vi "sub vi - password 1.vi"() -> (0 "RESULT":bool)   [LabVIEW 2013]
uses:
  program files/Global 1.vi
panel:
  in  "OK Button":bool
  in  "PASSWORD":string
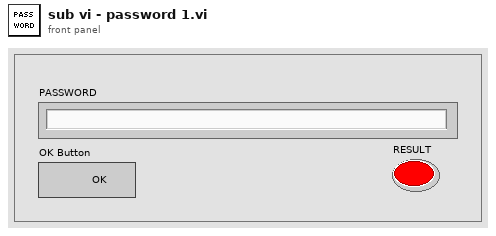
[diagram p1: front panel]
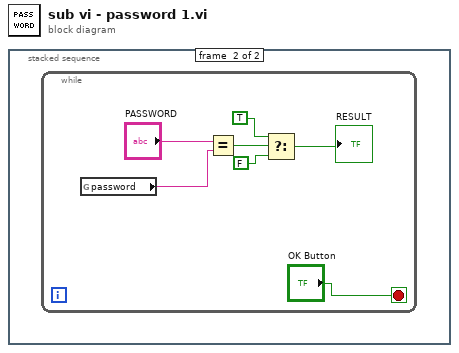
[diagram p0: block diagram]
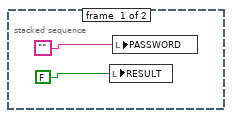
[diagram p2: hidden frame]
diagram:
  n1 = stacked-sequence {
    frame #0 {
      n2 = local write "RESULT"(FALSE) -> ()
      n3 = local write "PASSWORD"("") -> ()
    }
    frame #1 {
      n4 = while {
        stop <- "OK Button" stop-if-true
        n5 = global read "Global 1.vi" "password"() -> (w3:string)
        n6 = Equal?(x="PASSWORD", y=w3) -> (x = y?=w7:bool)
        n7 = Select(t=TRUE, s=w7, f=FALSE) -> (s? t:f=→"RESULT":bool)
      }
    }
  }
